vi "扫描脚本.vi"(8 "4-wire":bool, 10 "方向(T:正向)":bool=TRUE, 11 "扫描参数":T1={"+ V"=1.0, "+ Δ V"=0.01, "+ limit I"=0.01, "- V"=1.0, "- Δ V"=0.01, "- limit I"=0.01, "NPLC"=1.0, "模型"=FALSE} {"NPLC" min=0.001 max=25.0 step=0.001; "- Δ V" min=5e-05 max=1.0 step=5e-05 format="%#_6pV"; "+ Δ V" min=5e-05 max=1.0 step=5e-05 format="%#_6pV"; "- V" min=-40.0 max=40.0 format="%#_6pV"; "- limit I" min=1e-08 max=3.0 format="%#_6pA"; "+ limit I" min=1e-08 max=3.0 format="%#_6pA"; "+ V" min=-40.0 max=40.0 format="%#_6pV"}) -> (3 "Script":string)   [LabVIEW 2020, in "功能选择.xctl"]
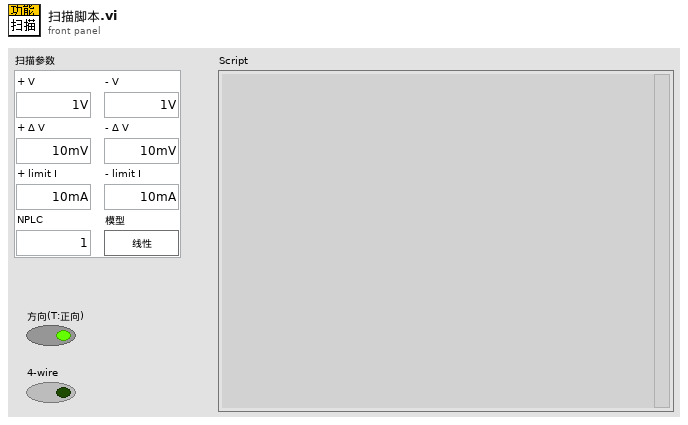
[diagram p1: front panel]
types:
  T1 = typedef "功能选择.xctl/扫描参数.ctl" = cluster{"+ V":dbl, "+ Δ V":dbl, "+ limit I":dbl, "- V":dbl, "- Δ V":dbl, "- limit I":dbl, "NPLC":dbl, "模型":bool}
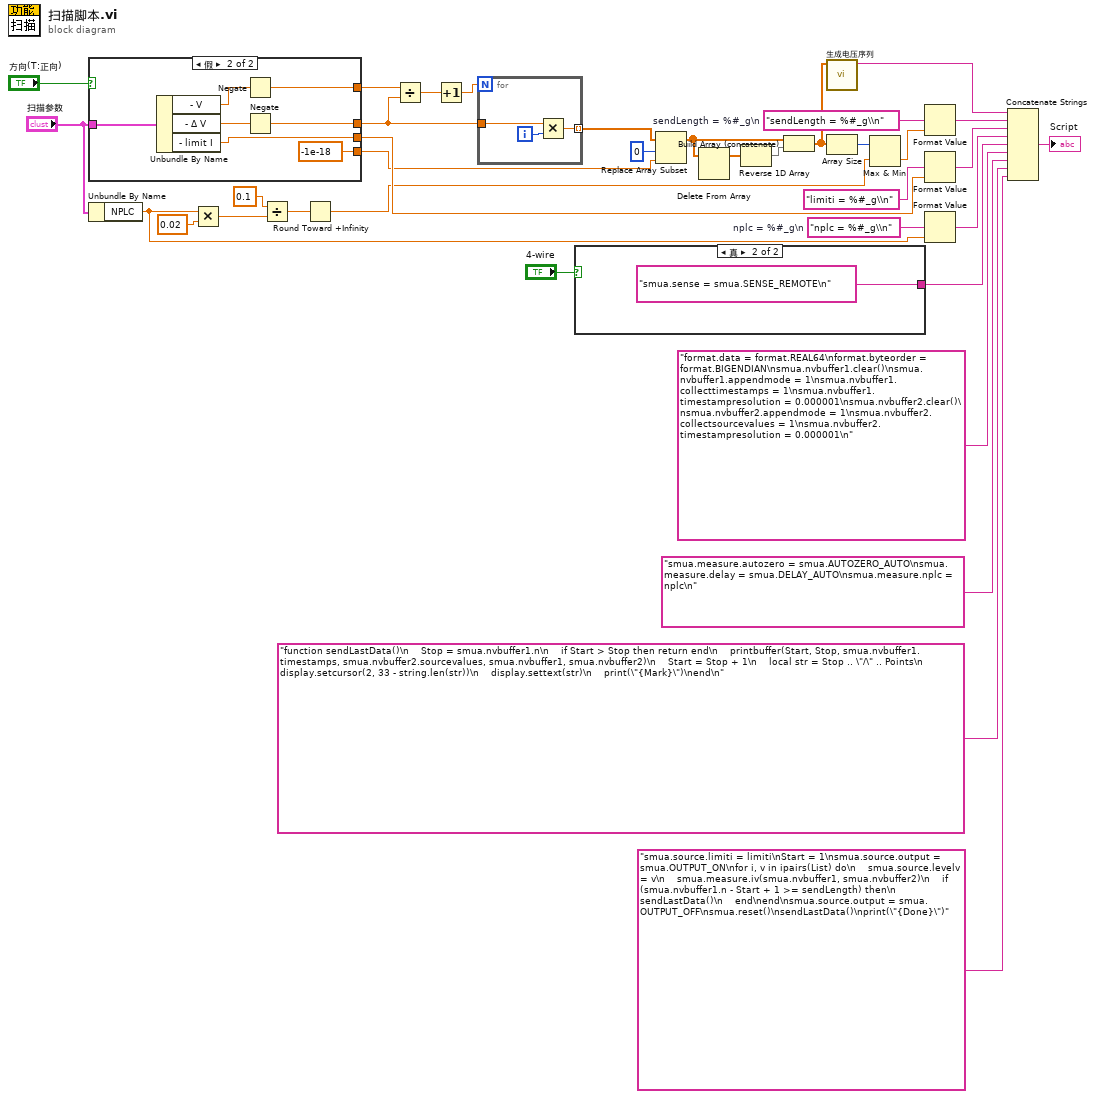
[diagram p0: block diagram]
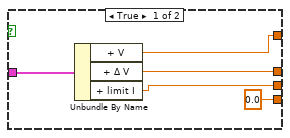
[diagram p2: hidden frame]
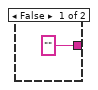
[diagram p3: hidden frame]
diagram:
  w22 = "nplc = %#_g\\n"  # nplc = %#_g\n
  w35 = "sendLength = %#_g\\n"  # sendLength = %#_g\n
  n1 = case shown="假" "方向(T:正向)" {
    tunnel: [w41 w47] -> w31
    tunnel: [w38 w43] -> w32
    tunnel: [w39 w46] -> w29
    tunnel: "扫描参数" -> [w40 w45]
    tunnel: [0.0 ("t") -1e-18 ("t")] -> w9
    frame True {
      n2 = Unbundle By Name(w40) -> ("+ V"=w41:dbl, "+ Δ V"=w39:dbl, "+ limit I"=w38:dbl)
    }
    frame False {
      n3 = Unbundle By Name(w45) -> ("- V"=w48:dbl, "- Δ V"=w44:dbl, "- limit I"=w43:dbl)
      n4 = Negate(x=w48) -> (-x=w47:dbl)
      n5 = Negate(x=w44) -> (-x=w46:dbl)
    }
  }
  n6 = Unbundle By Name("扫描参数") -> ("NPLC"=w21:dbl)
  n7 = Multiply(x=w21, y=0.02) -> (x*y=w18:dbl)
  n8 = Divide(x=0.1, y=w18) -> (x/y=w12:dbl)
  n9 = Round Toward +Infinity(x=w12) -> (ceil(x): smallest int >= x=w2:dbl)
  n10 = Divide(x=w31, y=w29) -> (x/y=w30:dbl)
  n11 = Increment(x=w30) -> (x+1=w26:dbl)
  n12 = for {
    N: w26 -> [_]
    tunnel: w29 -> [w50]
    tunnel: [w49] -> w25 mode=indexing
    i -> [w51]
    n13 = Multiply(x=w50, y=w51) -> (x*y=w49:dbl)
  }
  n14 = case shown="真" "4-wire" {
    tunnel: ["" "smua.sense = smua.SENSE_REMOTE\n"] -> w4
    frame False {
    }
    frame True {
    }
  }
  n15 = Replace Array Subset(array=w25, new element=w9, index=0 ("索引")) -> (w17:dbl[])
  n16 = Delete From Array(array=w17) -> (array with subset deleted=w27:dbl[])  [unwired: 2 in, 1 out]
  n17 = Reverse 1D Array(array=w27) -> (reversed array=w28:dbl[])
  n18 = Build Array (concatenate)(w17, w28) -> (w14:dbl[])
  n19 = call "生成电压序列.vi"("电压序列"=w14) -> ("List"=w24:string)  [unwired: 10 in]
  n20 = Array Size(array=w14) -> (size(s)=w13:i32)
  n21 = Max & Min(x=w13, y=w2) -> (min(x,y)=w11:dbl)  [unwired: 1 out]
  n22 = Format Value(format string=w35, value (0)=w11) -> (output string=w7:string)  [unwired: 1 in]
  n23 = Format Value(format string="limiti = %#_g\\n" ("格式字符串"), value (0)=w32) -> (output string=w6:string)  [unwired: 1 in]
  n24 = Format Value(format string=w22, value (0)=w21) -> (output string=w8:string)  [unwired: 1 in]
  n25 = Concatenate Strings(w24, w7, w6, w8, w4, "format.data = format.REAL64\nformat.byteorder = format.BIGENDIAN\nsmua.nvbuffer1.clear()\nsmua.nvbuffer1.appendmode = 1\nsmua.nvbuffer1.collecttimestamps = 1\nsmua.nvbuffer1.timestampresolution = 0.000001\nsmua.nvbuffer2.clear()\nsmua.nvbuffer2.appendmode = 1\nsmua.nvbuffer2.collectsourcevalues = 1\nsmua.nvbuffer2.timestampresolution = 0.000001\n", "smua.measure.autozero = smua.AUTOZERO_AUTO\nsmua.measure.delay = smua.DELAY_AUTO\nsmua.measure.nplc = nplc\n", "function sendLastData()\n    Stop = smua.nvbuffer1.n\n    if Start > Stop then return end\n    printbuffer(Start, Stop, smua.nvbuffer1.timestamps, smua.nvbuffer2.sourcevalues, smua.nvbuffer1, smua.nvbuffer2)\n    Start = Stop + 1\n    local str = Stop .. \"/\" .. Points\n    display.setcursor(2, 33 - string.len(str))\n    display.settext(str)\n    print(\"{Mark}\")\nend\n", "smua.source.limiti = limiti\nStart = 1\nsmua.source.output = smua.OUTPUT_ON\nfor i, v in ipairs(List) do\n    smua.source.levelv = v\n    smua.measure.iv(smua.nvbuffer1, smua.nvbuffer2)\n    if (smua.nvbuffer1.n - Start + 1 >= sendLength) then\n        sendLastData()\n    end\nend\nsmua.source.output = smua.OUTPUT_OFF\nsmua.reset()\nsendLastData()\nprint(\"{Done}\")") -> (→"Script":string)
